vi "Test Create Instrument SMO.vi"(8 "error in (no error)":errorcluster) -> (0 "error out":errorcluster)   [LabVIEW 2019]
uses:
  <vilib>/addons/_JKI Toolkits/Caraya/classes/Assert/Assert Not Error.vi
  <vilib>/addons/_JKI Toolkits/Caraya/classes/Assert/Assert.lvclass
  <vilib>/addons/_JKI Toolkits/Caraya/classes/Test/Test.lvclass
  lvsrc/Framework-Template/SMOs/Instrument.Framework-Template/Instrument.Framework-Template.lvclass
panel:
  # "1. Run This VI\n\n2. SMOs will start in \"debug\" mode.\n  --> Stop the Test Launcher that opens\n\n3. SMOs will run in normal mode.\n  --> Stop the Test Launcher that opens."
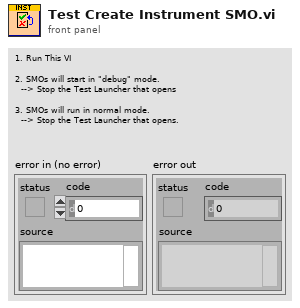
[diagram p1: front panel]
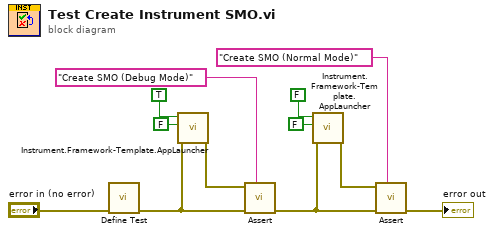
[diagram p0: block diagram]
diagram:
  n1 = call <vilib>:"Define Test.vi"("error in (no error)"="error in (no error)") -> ("error out"=w7:errorcluster)  [unwired: 9 in, 1 out]
  n2 = call "Instrument.Framework-Template.AppLauncher.vi"("error in"=w7, "Config Window"=FALSE ("Configuration Window? [T]"), "Debug Mode"=TRUE ("Debug Mode?")) -> ("error out"=w4:errorcluster)  [unwired: 8 in]
  n3 = call-poly <vilib>:"Assert.vi"("Label"="Create SMO (Debug Mode)", "error in (no error)"=w7, "Not Error?"=w4) -> ("error out"=w5:errorcluster)  [unwired: 7 in, 1 out]
  n4 = call "Instrument.Framework-Template.AppLauncher.vi"("error in"=w5, "Config Window"=FALSE ("Configuration Window? [T]"), "Debug Mode"=FALSE ("Debug Mode?")) -> ("error out"=w3:errorcluster)  [unwired: 8 in]
  n5 = call-poly <vilib>:"Assert.vi"("Label"="Create SMO (Normal Mode)", "error in (no error)"=w5, "Not Error?"=w3) -> ("error out"=→"error out":errorcluster)  [unwired: 7 in, 1 out]
